vi "I2C_flash_to_data.vi"(9 "Path":path, 10 "dwLen":u32, 11 "dwAddr":u32) -> (2 "data out":u8[](array[numeric]))   [LabVIEW 2016]
panel:
  in  "cmd_std_header_t":T1
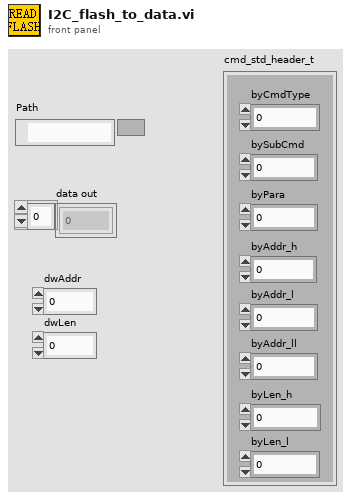
[diagram p1: front panel]
types:
  T1 = cluster{"byCmdType":u8, "bySubCmd":u8, "byPara":u8, "byAddr_h":u8, "byAddr_l":u8, "byAddr_ll":u8, "byLen_h":u8, "byLen_l":u8}
  T2 = enum16{"big-endian, network order", "native, host order", "little-endian"}
  T3 = enum16{"open", "replace", "create", "open or create", "replace or create", "replace or create with confirmation"}
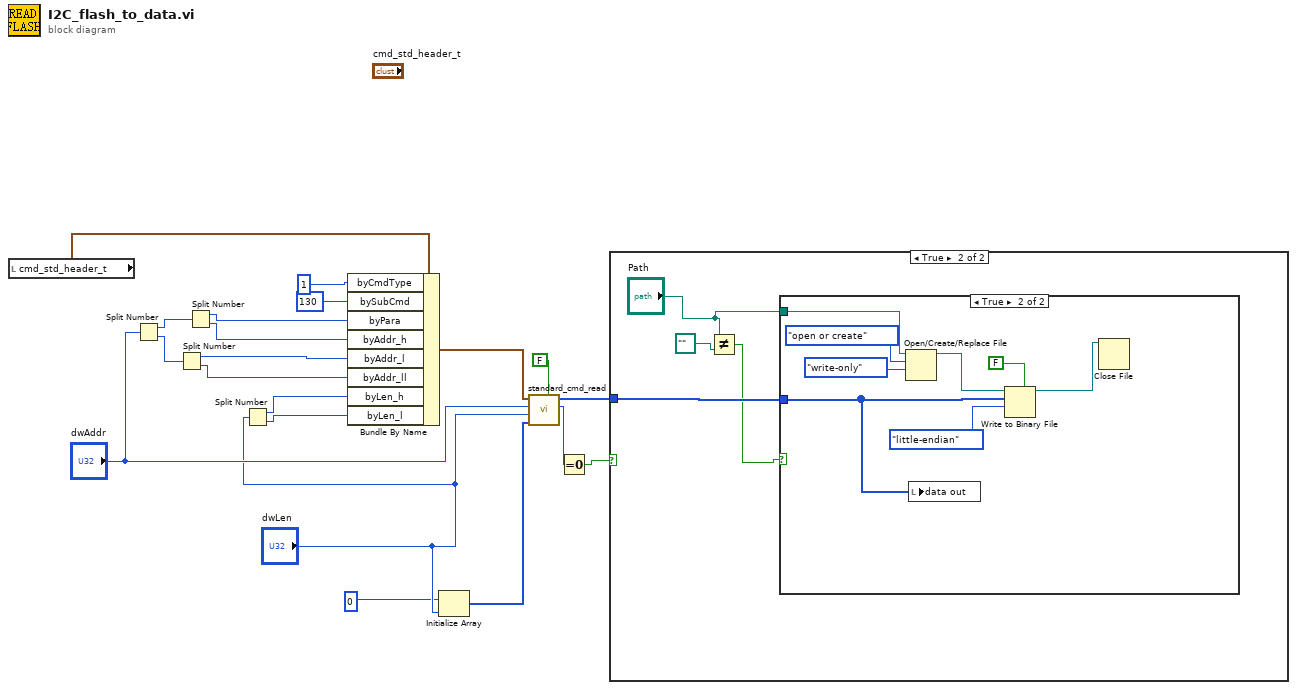
[diagram p0: block diagram]
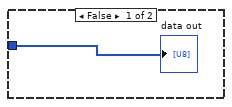
[diagram p3: hidden frame]
diagram:
  n1 = local read "cmd_std_header_t"() -> (w20:T1)
  n2 = Split Number(x="dwAddr") -> (hi(x)=w6:u16, lo(x)=w5:u16)
  n3 = Split Number(x=w5) -> (hi(x)=w10:u8, lo(x)=w9:u8)
  n4 = Split Number(x=w6) -> (hi(x)=w12:u8, lo(x)=w11:u8)
  n5 = Split Number(x="dwLen") -> (hi(x)=w8:u16, lo(x)=w7:u16)
  n6 = Bundle By Name(cluster=w20, "byCmdType"=u8 1, "bySubCmd"=u8 130, "byPara"=w12, "byAddr_h"=w11, "byAddr_l"=w10, "byAddr_ll"=w9, "byLen_h"=w8, "byLen_l"=w7) -> (w19:T1)
  n7 = Initialize Array(u8 0, "dwLen") -> (w2:u8[])
  n8 = call "standard_cmd_read.vi"("COM"=FALSE, "data"=w2, "dwLen"="dwLen", "dwAddr"="dwAddr", "cmd_std_header_t"=w19) -> ("return"=w13:i32, "data out"=w15:u8[])  [unwired: 4 in, 1 out]
  n9 = Equal To 0?(x=w13) -> (x = 0?=w14:bool)
  n10 = case shown="True" w14 {
    tunnel: w15 -> [_ w23]
    frame False {
    }
    frame True {
      n11 = Not Equal?(x="Path", y=path "") -> (x != y?=w21:bool)
      n12 = case shown="True" w21 {
        tunnel: w23 -> [w25 w26]
        tunnel: "Path" -> [_ w33]
        frame False {
          "data out" <- w25
        }
        frame True {
          n13 = Open/Create/Replace File(file path (use dialog)=w33, operation (0:open)=T3."open or create", access (0:read/write)=enum16{"read/write", "read-only", "write-only"}."write-only") -> (refnum out=w30:refnum<file>)  [unwired: 3 in, 2 out]
          n14 = local write "data out"(w26) -> ()
          n15 = Write to Binary File(file (use dialog)=w30, data=w26, 5:FALSE ("prepend array or string size? (T)"), 9:T2."little-endian" ("byte order (0:big-endian, network order)")) -> (refnum out=w28:refnum<file>)  [unwired: 2 in, 2 out]
          n16 = Close File(refnum=w28) -> ()  [unwired: 1 in, 2 out]
        }
      }
    }
  }
